vi "SourceGenerator.vi"(0 "method":enum16{"FileInput", "Direct"}(ring), 1 "file path":path=path "I:/05.0旅/非线性优化/Project/Simulation/abc.txt", 2 "AverageSize(bytes)":i32=500, 3 "SizeJitter(bytes)":i32=100, 4 "SourceQueue":refnum<queue>, 5 "Time Duration(ms)":u32(slide)=200 scale=0.0..500.0) -> (6 "size":i32, 8 "error out":errorcluster)   [LabVIEW 2014]
uses:
  <vilib>/Utility/tdmsutil.llb/TDMS Generate Random Data (U8).vi
panel:
  out "output cluster":T1
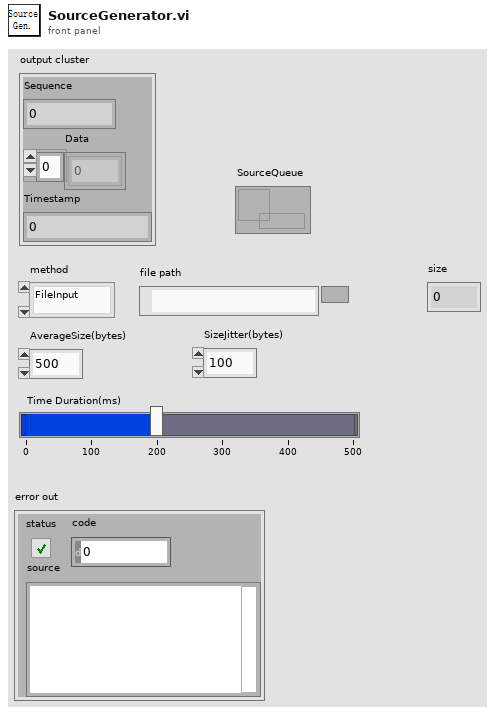
[diagram p1: front panel]
types:
  T1 = cluster{"Sequence":i32, "Data":u8[], "Timestamp":i32}
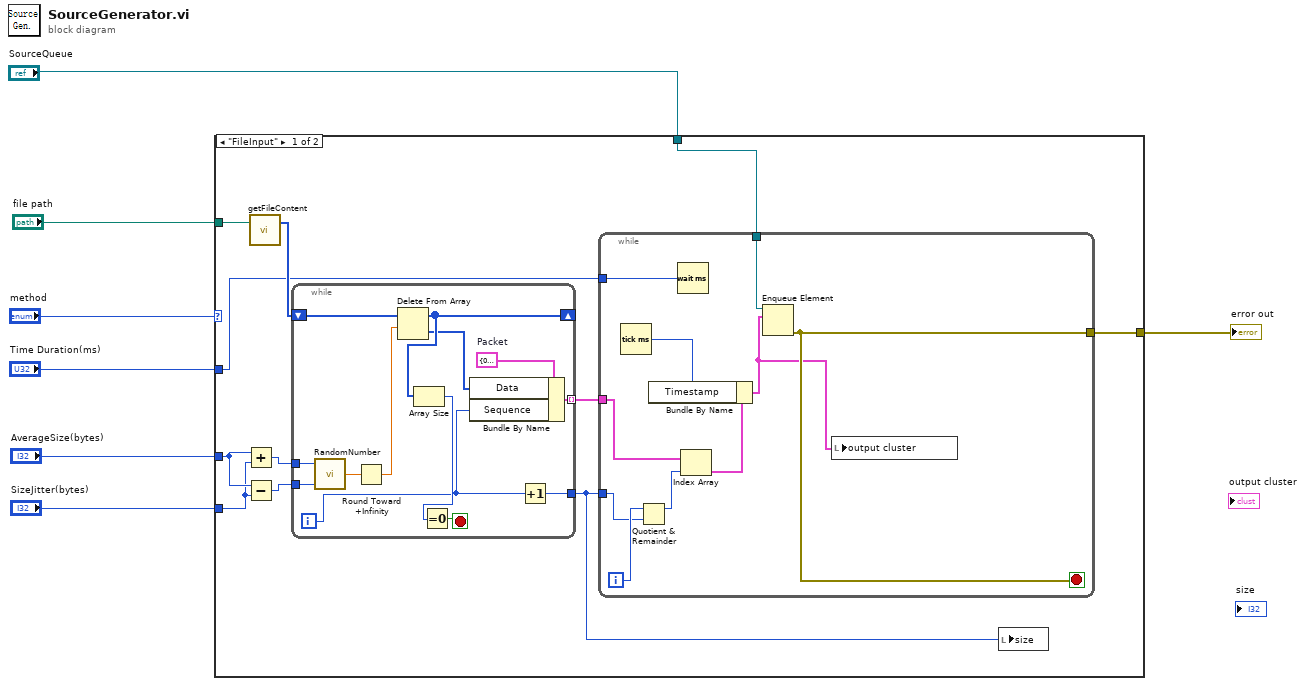
[diagram p0: block diagram]
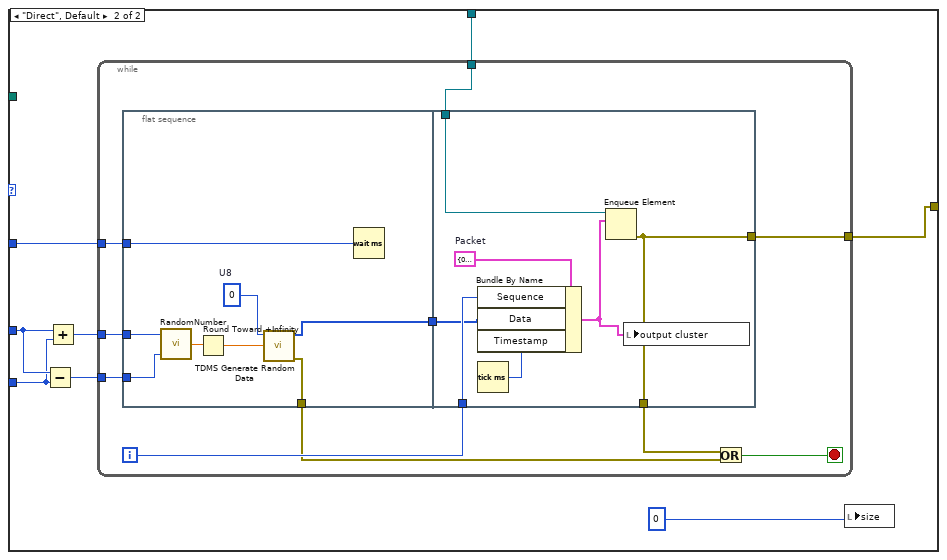
[diagram p2: hidden frame]
diagram:
  n1 = case shown="\"FileInput\"" "method" {
    tunnel: "file path" -> [w18 _]
    tunnel: "SourceQueue" -> [w8 w49]
    tunnel: "AverageSize(bytes)" -> [w16 w48]
    tunnel: "SizeJitter(bytes)" -> [w15 w47]
    tunnel: "Time Duration(ms)" -> [w11 w44]
    tunnel: [w9 w42] -> w2
    frame "FileInput" {
      n2 = Add(x=w16, y=w15) -> (x+y=w14:i32)
      n3 = Subtract(x=w16, y=w15) -> (x-y=w13:i32)
      n4 = call "getFileContent.vi"("file path"=w18) -> ("byte array"=w17:u8[])  [unwired: 1 in, 1 out]
      n5 = while {
        shift-right: [w36] -> _
        shift-left: w17 -> [w38]
        tunnel: w14 -> [w41]
        tunnel: w13 -> [w40]
        tunnel: [w32] -> w12 mode=indexing
        tunnel: [w30] -> w10
        i -> [w31]
        stop <- w35 stop-if-true
        w29 = T1 {"Sequence"=0, "Data"=[], "Timestamp"=0}  # Packet
        n6 = call "RandomNumber.vi"("Lower Bound"=w40, "Upper Bound"=w41) -> ("Value"=w39:dbl)  [unwired: 1 in]
        n7 = Round Toward +Infinity(x=w39) -> (ceil(x): smallest int >= x=w37:dbl)
        n8 = Delete From Array(array=w38, length=w37) -> (deleted portion=w33:u8[], array with subset deleted=w36:u8[])  [unwired: 1 in]
        n9 = Array Size(array=w36) -> (size(s)=w34:i32)
        n10 = Equal To 0?(x=w34) -> (x = 0?=w35:bool)
        n11 = Bundle By Name(cluster=w29, "Data"=w33, "Sequence"=w31) -> (w32:T1)
        n12 = Increment(x=w31) -> (x+1=w30:i32)
      }
      n13 = while {
        tunnel: w12 -> [w21]
        tunnel: w10 -> [w26]
        tunnel: w11 -> [w28]
        tunnel: [w24] -> w9
        tunnel: w8 -> [w23]
        i -> [w27]
        stop <- w24 stop-if-true
        n14 = Tick Count (ms)() -> (millisecond timer value=w22:u32)
        n15 = Quotient & Remainder(x=w27, y=w26) -> (x-y*floor(x/y)=w25:i32)  [unwired: 1 out]
        n16 = Wait (ms)(milliseconds to wait=w28) -> ()  [unwired: 1 out]
        n17 = Index Array(array=w21, index=w25) -> (element=w20:T1)
        n18 = Bundle By Name(cluster=w20, "Timestamp"=w22) -> (w19:T1)
        n19 = Enqueue Element(queue=w23, element=w19) -> (error out=w24:errorcluster)  [unwired: 2 in, 2 out]
        n20 = local write "output cluster"(w19) -> ()
      }
      n21 = local write "size"(w10) -> ()
    }
    frame "Direct", Default {
      n22 = Subtract(x=w48, y=w47) -> (x-y=w45:i32)
      n23 = Add(x=w48, y=w47) -> (x+y=w46:i32)
      n24 = while {
        tunnel: w49 -> [w59]
        tunnel: w46 -> [w53]
        tunnel: w45 -> [w52]
        tunnel: w44 -> [w51]
        tunnel: [w50] -> w42
        i -> [w58]
        stop <- w54 stop-if-true
        n25 = flat-sequence {
          tunnel: [w64] -> w57
          tunnel: [w63] -> w55
          tunnel: w53 -> [w62]
          tunnel: w52 -> [w61]
          tunnel: w51 -> [w60]
          tunnel: w59 -> [w72]
          tunnel: w58 -> [w74]
          tunnel: w57 -> [w73]
          tunnel: [w71] -> w56
          tunnel: [w71] -> w50
          frame #0 {
            w66 = u8 0  # U8
            n26 = call "RandomNumber.vi"("Lower Bound"=w61, "Upper Bound"=w62) -> ("Value"=w67:dbl)  [unwired: 1 in]
            n27 = Round Toward +Infinity(x=w67) -> (ceil(x): smallest int >= x=w65:dbl)
            n28 = call-poly <vilib>:"TDMS Generate Random Data.vi"("number of samples"=w65, "data type"=w66) -> ("error out"=w63:errorcluster, "data"=w64:u8[])  [unwired: 8 in]
            n29 = Wait (ms)(milliseconds to wait=w60) -> ()  [unwired: 1 out]
          }
          frame #1 {
            w70 = T1 {"Sequence"=0, "Data"=[], "Timestamp"=0}  # Packet
            n30 = Tick Count (ms)() -> (millisecond timer value=w69:u32)
            n31 = Bundle By Name(cluster=w70, "Sequence"=w74, "Data"=w73, "Timestamp"=w69) -> (w68:T1)
            n32 = Enqueue Element(queue=w72, element=w68) -> (error out=w71:errorcluster)  [unwired: 2 in, 2 out]
            n33 = local write "output cluster"(w68) -> ()
          }
        }
        n34 = Or(x=w56, y=w55) -> (x .or. y?=w54:bool)
      }
      n35 = local write "size"(0) -> ()
    }
  }
  "error out" <- w2
